vi "Harv_2_9.vi"(0 "HarvSetpoints":dbl[](array[numeric]), 1 "HarvPot":dbl, 3 "Count":i32, 4 "BallAcquired":bool, 5 "FireBallSen":bool, 6 "Fire":bool, 7 "Harvest":bool, 8 "HPButton":bool, 9 "inAuton?":bool, 10 "WinchDown":bool, 11 "AutonMoved":bool, 12 "HarvPivUP":bool, 13 "HarvPivPickupLim":bool) -> (14 "HarvPower":dbl, 15 "HarvRoller":dbl, 16 "AutonReadyToMove":bool, 17 "CountOut":i32, 18 "HarvStart":bool, 19 "HarvCleared":bool)   [LabVIEW 2013]
panel:
  in  "MotorScale":dbl=1.5
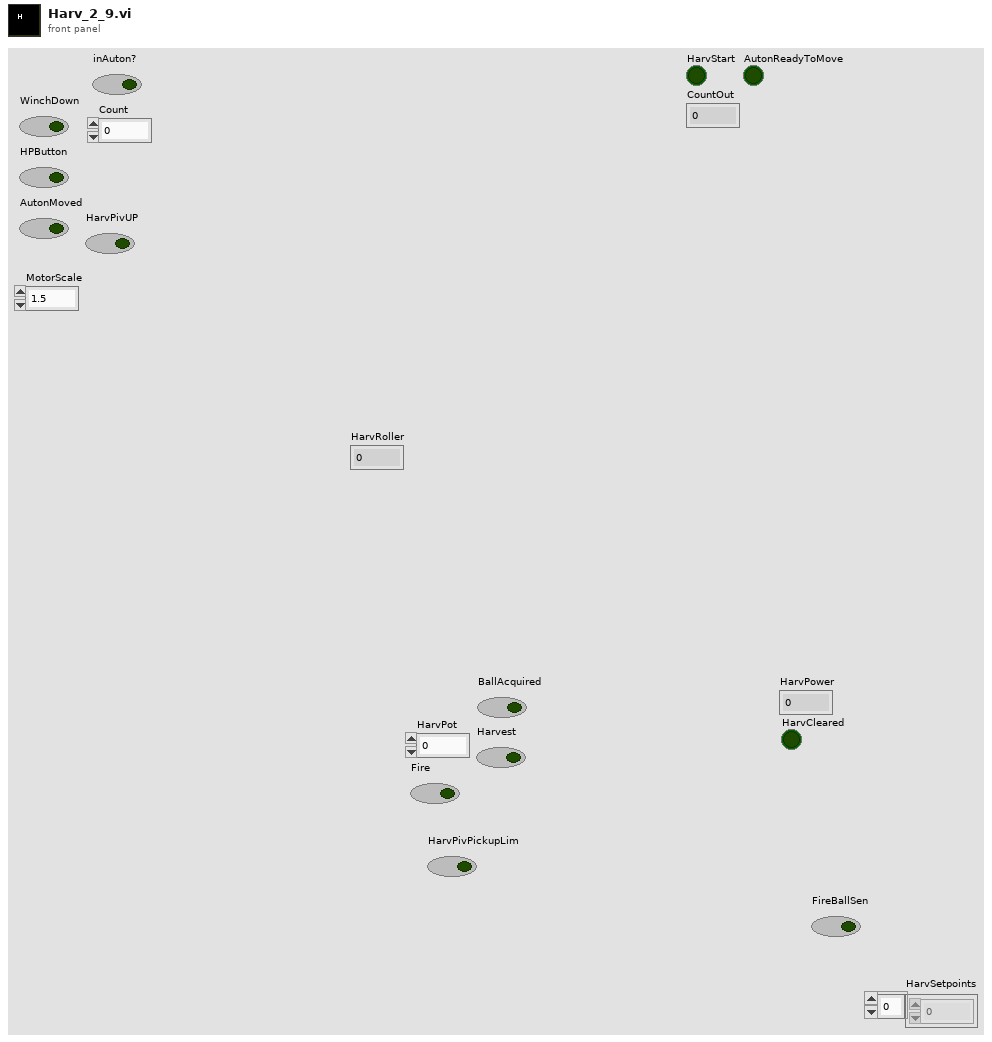
[diagram p1: front panel]
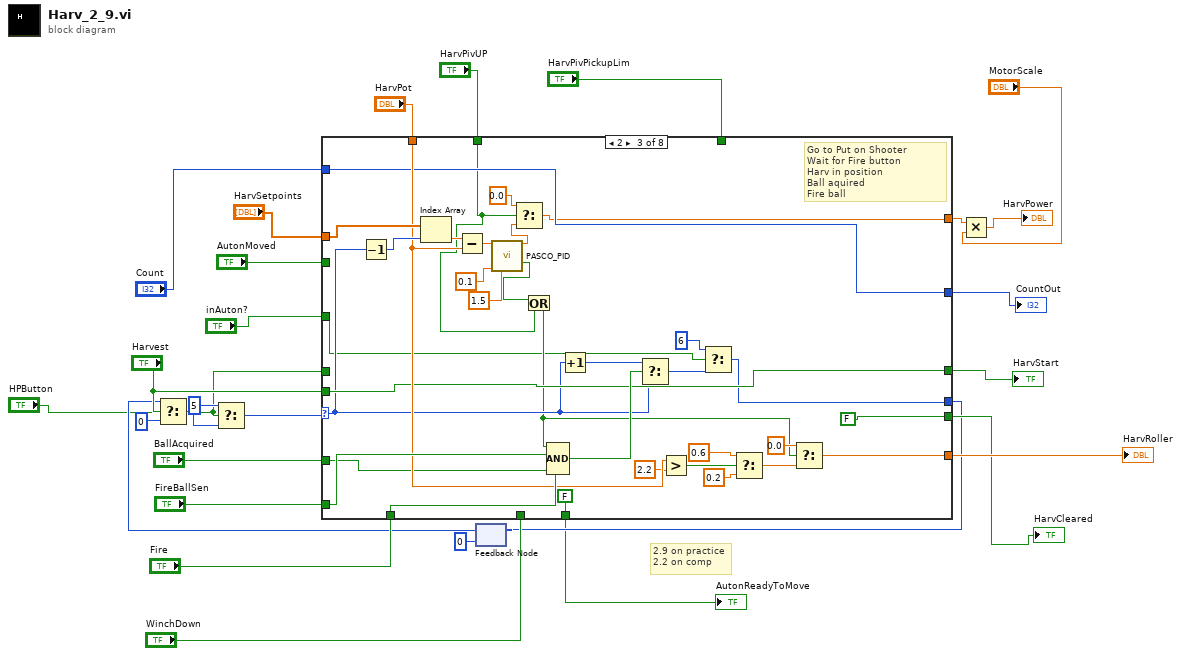
[diagram p0: block diagram]
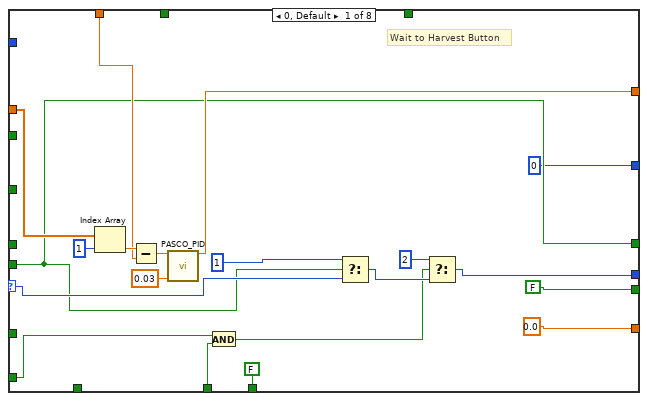
[diagram p2: hidden frame]
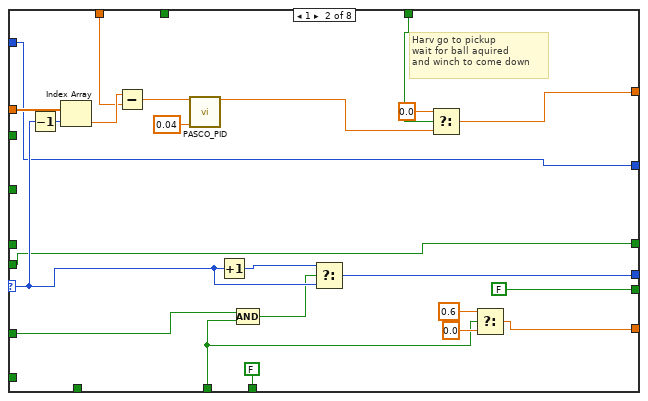
[diagram p3: hidden frame]
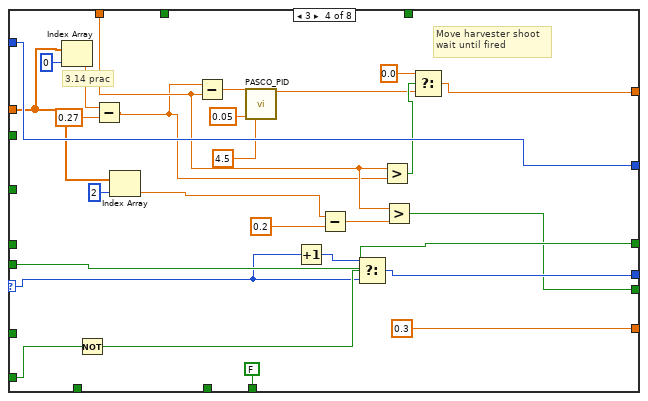
[diagram p4: hidden frame]
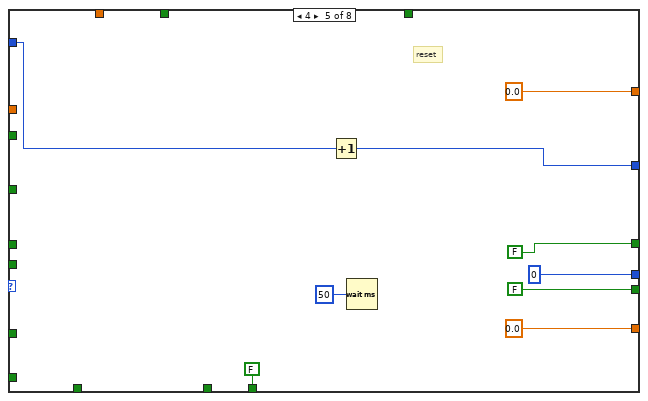
[diagram p5: hidden frame]
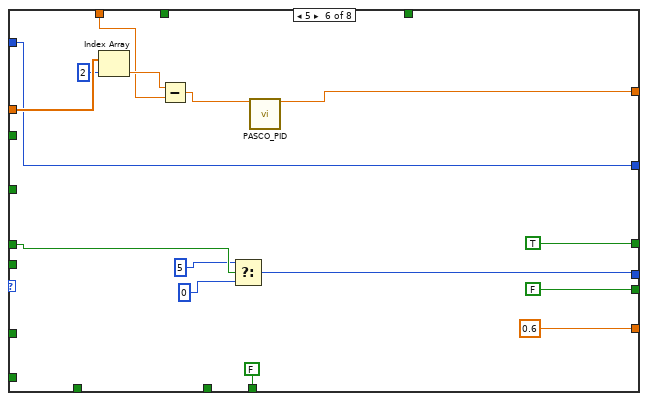
[diagram p6: hidden frame]
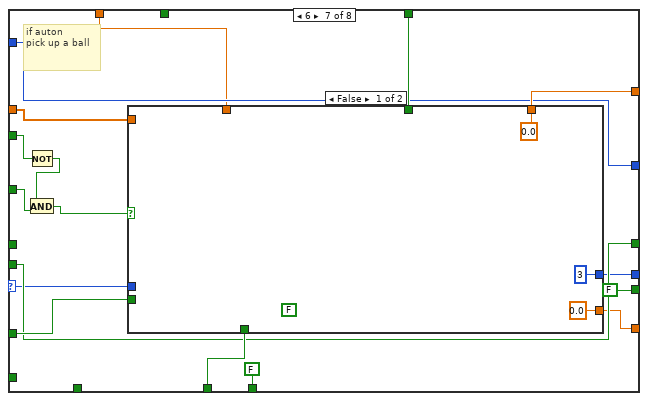
[diagram p7: hidden frame]
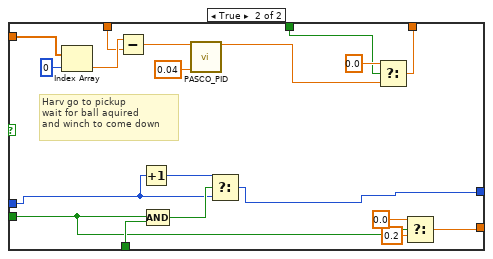
[diagram p8: hidden frame]
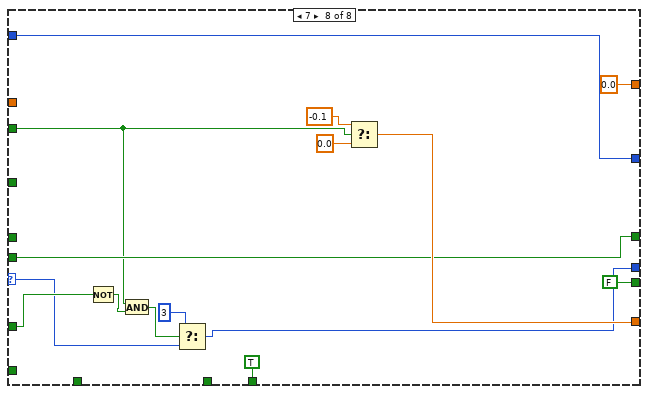
[diagram p9: hidden frame]
diagram:
  # "2.9 on practice\n2.2 on comp"
  n1 = feedback #1(0 ("f")) -> (w21:i32)
  n2 = Select(t=w21, s="Harvest", f=0) -> (s? t:f=w6:i32)
  n3 = Select(t=5, s="HPButton", f=w6) -> (s? t:f=w5:i32)
  n4 = case shown="2" w5 {
    selector: w5 -> [w45 w64 w85 w125 _ _ w165 w199]
    tunnel: "HarvSetpoints" -> [w44 w71 w105 w110 _ w156 w172 _]
    tunnel: "HarvPot" -> [w43 w69 w97 w115 _ w153 w159 _]
    tunnel: [w38 w51 w72 w117 0.0 ("Output") w151 w171 0.0 ("Output")] -> w20
    tunnel: [w35 w66 w75 w130 0 ("t") w146 w166 w198] -> w10
    tunnel: [0.0 ("f") w58 w90 0.3 ("f") 0.0 ("f") 0.6 ("f") w167 w207] -> w26
    tunnel: "BallAcquired" -> [_ w60 w87 _ _ _ w169 w203]
    tunnel: "FireBallSen" -> [w33 _ w101 w128 _ _ _ _]
    tunnel: "Fire" -> [_ _ w100 _ _ _ _ _]
    tunnel: "Harvest" -> [w36 w61 w88 w129 _ _ w168 w204]
    tunnel: [FALSE ("IsThere") FALSE ("IsThere") FALSE ("IsThere") w116 FALSE ("IsThere") FALSE ("IsThere") FALSE ("IsThere") FALSE ("IsThere")] -> w17
    tunnel: "HarvPivPickupLim" -> [_ w53 _ _ _ _ w173 _]
    tunnel: "HarvPivUP" -> [_ _ w80 _ _ _ _ _]
    tunnel: [w36 w61 w88 w129 FALSE ("Harvest") TRUE ("Harvest") w168 w204] -> w14
    tunnel: "WinchDown" -> [w32 w55 _ _ _ _ w170 _]
    tunnel: "inAuton?" -> [_ _ w73 _ _ _ w160 _]
    tunnel: [0 ("Count") w54 w84 w124 w135 w150 w164 w209] -> w8
    tunnel: "Count" -> [_ w54 w84 w124 w134 w150 w164 w209]
    tunnel: "HPButton" -> [_ _ _ _ _ w149 _ _]
    tunnel: [FALSE FALSE FALSE FALSE FALSE FALSE FALSE TRUE] -> w2
    tunnel: "AutonMoved" -> [_ _ _ _ _ _ w158 w202]
    frame 0, Default {
      # "Wait to Harvest Button"
      n5 = Index Array(array=w44, index=1) -> (element=w46:dbl)
      n6 = Subtract(x=w46, y=w43) -> (x-y=w47:dbl)
      n7 = call "PASCO_PID.vi"("Delta"=w47, "Deadband"=0.03) -> ("Output"=w38:dbl)  [unwired: 12 in, 1 out]
      n8 = And(x=w33, y=w32) -> (x .and. y?=w31:bool)
      n9 = Select(t=1, s=w36, f=w45) -> (s? t:f=w37:i32)
      n10 = Select(t=2, s=w31, f=w37) -> (s? t:f=w35:i32)
    }
    frame 1 {
      # "Harv go to pickup\nwait for ball aquired\nand winch to come down"
      n11 = Decrement(x=w64) -> (x-1=w65:i32)
      n12 = Index Array(array=w71, index=w65) -> (element=w70:dbl)
      n13 = Subtract(x=w70, y=w69) -> (x-y=w68:dbl)
      n14 = call "PASCO_PID.vi"("Delta"=w68, "Deadband"=0.04) -> ("Output"=w52:dbl)  [unwired: 12 in, 1 out]
      n15 = Increment(x=w64) -> (x+1=w67:i32)
      n16 = Compound Arithmetic op=AND(w60, w55) -> (w59:bool)
      n17 = Select(t=w67, s=w59, f=w64) -> (s? t:f=w66:i32)
      n18 = Select(t=0.0, s=w53, f=w52) -> (s? t:f=w51:dbl)
      n19 = Select(t=0.6, s=w55, f=0.0) -> (s? t:f=w58:dbl)
    }
    frame 2 {
      # "Go to Put on Shooter\nWait for Fire button\nHarv in position\nBall aquired \nFire ball"
      n20 = Decrement(x=w85) -> (x-1=w99:i32)
      n21 = Index Array(array=w105, index=w99) -> (element=w104:dbl)
      n22 = Subtract(x=w104, y=w97) -> (x-y=w103:dbl)
      n23 = call "PASCO_PID.vi"("Delta"=w103, "Deadband"=0.1, "P Gain"=1.5) -> ("Output"=w83:dbl, "IsThere"=w81:bool)  [unwired: 11 in]
      n24 = Select(t=0.0, s=w80, f=w83) -> (s? t:f=w72:dbl)
      n25 = Or(x=w81, y=w80) -> (x .or. y?=w79:bool)
      n26 = Compound Arithmetic op=AND(w79, w101, w100, w87) -> (w102:bool)
      n27 = Increment(x=w85) -> (x+1=w86:i32)
      n28 = Select(t=w86, s=w102, f=w85) -> (s? t:f=w76:i32)
      n29 = Greater?(x=w97, y=2.2) -> (0:w95:bool)
      n30 = Select(t=6, s=w73, f=w76) -> (s? t:f=w75:i32)
      n31 = Select(t=0.6, s=w95, f=0.2) -> (s? t:f=w91:dbl)
      n32 = Select(t=0.0, s=w79, f=w91) -> (s? t:f=w90:dbl)
    }
    frame 3 {
      # "3.14 prac"
      # "Move harvester shoot\nwait until fired"
      n33 = Index Array(array=w110, index=0) -> (element=w109:dbl)
      n34 = Not(x=w128) -> (.not. x?=w127:bool)
      n35 = Subtract(x=w109, y=0.27) -> (x-y=w108:dbl)
      n36 = Index Array(array=w110, index=2) -> (element=w113:dbl)
      n37 = Subtract(x=w108, y=w115) -> (x-y=w123:dbl)
      n38 = call "PASCO_PID.vi"("Delta"=w123, "Deadband"=0.05, "P Gain"=4.5) -> ("Output"=w118:dbl)  [unwired: 11 in, 1 out]
      n39 = Increment(x=w125) -> (x+1=w126:i32)
      n40 = Subtract(x=w113, y=0.2) -> (x-y=w114:dbl)
      n41 = Select(t=w126, s=w127, f=w125) -> (s? t:f=w130:i32)
      n42 = Greater?(x=w115, y=w108) -> (0:w120:bool)
      n43 = Greater?(x=w115, y=w114) -> (0:w116:bool)
      n44 = Select(t=0.0, s=w120, f=w118) -> (s? t:f=w117:dbl)
    }
    frame 4 {
      # "reset"
      n45 = Increment(x=w134) -> (x+1=w135:i32)
      n46 = Wait (ms)(milliseconds to wait=u32 50) -> ()  [unwired: 1 out]
    }
    frame 5 {
      n47 = Index Array(array=w156, index=2) -> (element=w154:dbl)
      n48 = Subtract(x=w154, y=w153) -> (x-y=w152:dbl)
      n49 = Select(t=5 ("index"), s=w149, f=0 ("index")) -> (s? t:f=w146:i32)
      n50 = call "PASCO_PID.vi"("Delta"=w152) -> ("Output"=w151:dbl)  [unwired: 13 in, 1 out]
    }
    frame 6 {
      # "if auton \npick up a ball"
      n51 = Not(x=w158) -> (.not. x?=w157:bool)
      n52 = And(x=w157, y=w160) -> (x .and. y?=w161:bool)
      n53 = case shown="False" w161 {
        tunnel: w173 -> [_ w191]
        tunnel: w172 -> [_ w190]
        tunnel: [0.0 ("Output") w187] -> w171
        tunnel: w170 -> [_ w186]
        tunnel: w169 -> [_ w184]
        tunnel: [0.0 ("f") w185] -> w167
        tunnel: [3 w180] -> w166
        tunnel: w165 -> [_ w178]
        tunnel: w159 -> [_ w177]
        frame False {
          (unwired) FALSE
        }
        frame True {
          # "Harv go to pickup\nwait for ball aquired\nand winch to come down"
          n54 = Index Array(array=w190, index=0) -> (element=w189:dbl)
          n55 = Subtract(x=w189, y=w177) -> (x-y=w192:dbl)
          n56 = Increment(x=w178) -> (x+1=w179:i32)
          n57 = Compound Arithmetic op=AND(w184, w186) -> (w181:bool)
          n58 = call "PASCO_PID.vi"("Delta"=w192, "Deadband"=0.04) -> ("Output"=w194:dbl)  [unwired: 12 in, 1 out]
          n59 = Select(t=w179, s=w181, f=w178) -> (s? t:f=w180:i32)
          n60 = Select(t=0.0, s=w191, f=w194) -> (s? t:f=w187:dbl)
          n61 = Select(t=0.0, s=w184, f=0.2) -> (s? t:f=w185:dbl)
        }
      }
    }
    frame 7 {
      n62 = Not(x=w203) -> (.not. x?=w201:bool)
      n63 = And(x=w202, y=w201) -> (x .and. y?=w200:bool)
      n64 = Select(t=3, s=w200, f=w199) -> (s? t:f=w198:i32)
      n65 = Select(t=-0.1, s=w202, f=0.0) -> (s? t:f=w207:dbl)
    }
  }
  "HarvRoller" <- w26
  "HarvCleared" <- w17
  "HarvStart" <- w14
  "CountOut" <- w8
  "AutonReadyToMove" <- w2
  n66 = feedback-in #1(w10) -> ()
  n67 = Multiply(x=w20, y="MotorScale") -> (x*y=→"HarvPower":dbl)
